vi "华为UPS2000-G-(1-3KVA)界面.vi"() -> ()   [LabVIEW 2016, in "环境动力监测库.lvlib" / "UPS库.lvlib"]
panel:
  out "Port":string
  out "IP":string
  out "x+1":u32
  in  "解除告警":bool
  out "通信":bool=TRUE
  out "串口":string
  in  "停止自检":bool
  in  "启动自检":bool
  out "UPS状态":T1
  out "电池状态":T2 {"电池状态" items=["休眠"=2, "浮充"=3, "均充"=4, "放电"=5]}
  out "UPS参数":T3 {"开机状态" items=["关机", "开机中", "开机失败", "开机完成"]}
  in  "查看型号":bool
  in  "重开串口":bool
  # "V"
  # "%"
  # "S"
  # "Ah"
  # "kVA"
  # "V"
  # "Hz"
  # "V"
  # "A"
  # "Hz"
  # "kW"
  # "kVA"
  # "%"
  # "℃"
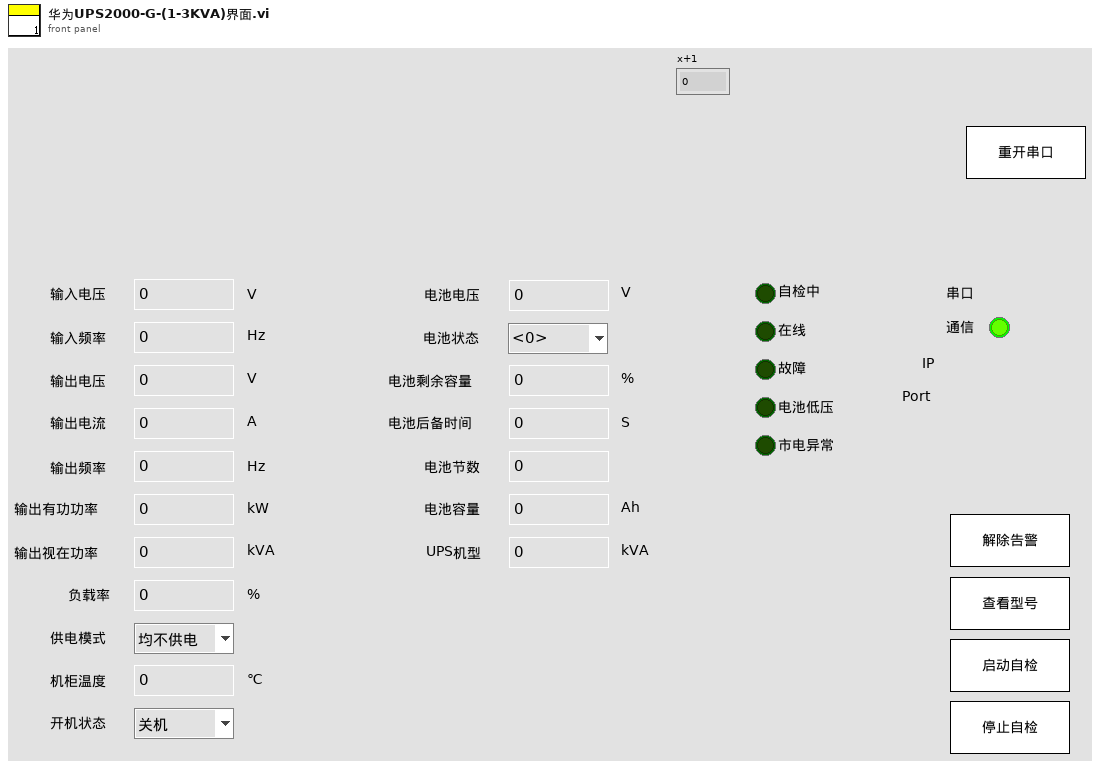
[diagram p1: front panel]
types:
  T1 = cluster{"保留":bool, "保留":bool, "自检中":bool, "在线":bool, "故障":bool, "保留":bool, "电池低压":bool, "市电异常":bool}
  T2 = cluster{"电池电压":dbl, "电池状态":u16, "电池剩余容量":u16, "电池后备时间":u32, "电池节数":u16, "电池容量":u16, "UPS机型":u16}
  T3 = cluster{"输入电压":dbl, "输入频率":dbl, "旁路电压V":dbl, "旁路频率HZ":dbl, "输出电压":dbl, "输出电流":dbl, "输出频率":dbl, "输出有功功率":dbl, "输出视在功率":dbl, "负载率":dbl, "供电模式":enum16{"均不供电", "旁路供电", "主路供电", "电池供电", "主路ECO"}, "输入制式0:单相":u16, "输出制式0:单相":u16, "机柜温度":dbl, "开机状态":u16, "UPS状态":u8}
  T4 = typedef "环境动力监测库.lvlib/UPS库.lvlib/UPS型号.ctl" = enum16{"山特UPSC1~3", "山特UPSC6~20", "华为UPS2000-G-(1-3KVA)", "Kstar"}
  T5 = cluster{"VISA resource name":refnum<visa-resource-name>, "Serial Config":cluster{"baud rate (9600)":u32, "stop bits (10: 1 bit)":u16, "parity (0:none)":enum16{"None", "Odd", "Even", "Mark", "Space"}, "data bits (8)":u16, "timeout (10sec)":u32}, "型号选择":T4, "HW-UPS-2000 MB session":refnum<class "MB_Master.lvclass">, "连接方式":enum16{"串口", "TCP"}, "IP":string, "Port":string, "低电量报警阈值":u16, "功能启用":bool}
  T6 = cluster{"输入电压V":dbl, "输入频率HZ":dbl, "旁路电压V":dbl, "旁路频率HZ":dbl, "输出电压V":dbl, "输出电流A":dbl, "输出频率HZ":dbl, "输出有功功率kW":dbl, "输出视在功率kVA":dbl, "负载率%":dbl, "供电模式":enum16{"均不供电", "旁路供电", "主路供电", "电池供电", "主路ECO"}, "输入制式0:单相":u16, "输出制式0:单相":u16, "机柜温度℃":dbl, "开机状态":u16, "UPS状态":u8}
  T7 = cluster{"电池电压V":dbl, "电池状态":u16, "电池剩余容量%":u16, "电池后备时间s":u32, "电池节数":u16, "电池容量AH":u16, "UPS机型KVA":u16}
  T8 = cluster{"市电":cluster{"状态":bool, "电压:":u16, "电流：":dbl, "详情  ":bool}, "UPS":cluster{"状态":bool, "输入电压:":sgl, "输出电压:":sgl, "电池电量:":u8, "电量":u16, "详情  ":bool}, "蓄电池12V":cluster{"状态":bool, "电压:":sgl, "电流:":sgl, "电池电量:":u8, "电量":u16, "详情  ":bool, "充电":bool, "负载":bool}, "蓄电池24V":cluster{"状态":bool, "电压:":sgl, "电流:":sgl, "电池电量:":u8, "电量":u16, "详情  ":bool, "充电":bool, "负载":bool}}
  T9 = cluster{"华为2000-G-UPS状态[0]":bool, "华为2000-G-UPS状态[1]":bool, "华为2000-G-UPS状态[2]":bool, "华为2000-G-UPS状态[3]":bool, "华为2000-G-UPS状态[4]":bool, "华为2000-G-UPS状态[5]":bool, "华为2000-G-UPS状态[6]":bool, "华为2000-G-UPS状态[7]":bool}
  T10 = enum32{"Bad", "Idle", "Run top level", "Running"}
  T11 = cluster{"漏水监测输出":cluster{"漏水监测告警":bool, "告警内容":string}, "门禁监测输出":cluster{"门禁监测告警":bool, "告警内容":string}, "门禁监测输出2":cluster{"门禁监测告警":bool, "告警内容":string}, "温湿度监测输出":cluster{"温湿度监测告警":bool, "告警内容":string}, "烟雾监测输出":cluster{"烟雾监测告警":bool, "告警内容":string}, "空调监测输出":cluster{"空调监测告警":bool, "告警内容":string}, "自动重合闸输出":cluster{"自动重合闸告警":bool, "告警内容":string}, "红外入侵输出":cluster{"红外入侵告警":bool, "告警内容":string}, "振动输出":cluster{"振动告警":bool, "告警内容":string}, "UPS输出":cluster{"UPS告警":bool, "告警内容":string}, "蓄电池输出":cluster{"蓄电池告警":bool, "告警内容":string}, "蓄电池输出2":cluster{"蓄电池告警":bool, "告警内容":string}, "GPS输出":cluster{"定位告警":bool, "告警内容":string}, "北斗输出":cluster{"定位告警":bool, "告警内容":string}, "气象输出":cluster{"气象告警":bool, "告警内容":string}, "废液输出":cluster{"废液告警":bool, "告警内容":string}, "废液输出2":cluster{"废液告警":bool, "告警内容":string}, "灭火装置输出":cluster{"灭火装置告警":bool, "告警内容":string}}
  T12 = typedef "工况数据.ctl" = cluster{"time":string, "data":cluster{"ups":cluster{"ups":cluster{"input_voltage":ext, "input_frequency":ext, "output_voltage":ext, "output_current":ext, "output_frequency":ext, "output_active_power":ext, "output_apparent_power":ext, "load_rate":ext, "cabinet_temperature":ext, "battery_voltage":ext, "remaining_battery_capacity":ext, "power_on_status":string, "power_supply_mode":string, "fault":bool, "battery_low_voltage":bool, "mains_supply_abnormality":bool}, "启用":bool}, "air_conditioner":cluster{"air_conditioner":cluster{"cabinet_temperature":ext, "air_supply_temperature":ext, "voltage":ext, "current":ext, "compressor_status":string, "Internal_fan_status":string, "external_fan_status":string, "heating_state":string, "refrigeration_state":bool, "high_temperature_alarm":bool, "low_temperature_alarm":bool, "heater_fault":bool, "temperature_sensor_fault":bool, "high_voltage_alarm":bool, "low_voltage_alarm":bool, "refrigeration_start_point":ext, "refrigeration_sensitive_point":ext, "heating_start_point":ext, "heating_sensitive_point":ext, "high_temperature_alarm_point":ext, "low_temperature_alarm_point":ext}, "启用":bool}, "smoke_sensor":cluster{"smoke_sensor":cluster{"trigger_alarm":bool}, "启用":bool}, "water_immersion_sensor":cluster{"water_immersion_sensor":cluster{"trigger_alarm":bool}, "启用":bool}, "temperature_and_humidity_sensor":cluster{"temperature_and_humidity_sensor":cluster{"current_temperature":ext, "current_humidity":ext, "room_temperature_alarm":bool, "humidity_alarm":bool}, "启用":bool}, "gps":cluster{"gps":cluster{"current_longitude":ext, "current_latitude":ext, "launch_longitude":ext, "launch_latitude":ext, "shift_alarm":bool}, "启用":bool}, "solar_controller":cluster{"solar_controller":cluster{"array_voltage":ext, "array_current":ext, "generating_power":ext, "battery_voltage":dbl, "battery_current":ext, "ceiling_voltage":ext, "minimum_voltage":ext, "battery_temperature":ext, "remaining_battery_capacity":ext, "load_voltage":ext, "load_current":ext, "load_power":ext, "equipment_temperature":ext, "accumulated_electricity_consumption_of_the_day":ext, "accumulated_electricity_consumption_of_the_current_month":ext, "accumulated_electricity_consumption_in_the_current_year":ext, "total_accumulated_power_consumption":ext, "accumulated_charging_capacity_of_the_day":ext, "accumulated_charging_amount_of_the_current_month":ext, "accumulated_charging_capacity_of_the_current_year":ext, "total_cumulative_charge":ext}, "启用":bool}, "solar_controller_2":cluster{"solar_controller_2":cluster{"array_voltage":ext, "array_current":ext, "generating_power":ext, "battery_voltage":dbl, "battery_current":ext, "ceiling_voltage":ext, "minimum_voltage":ext, "battery_temperature":ext, "remaining_battery_capacity":ext, "load_voltage":ext, "load_current":ext, "load_power":ext, "equipment_temperature":ext, "accumulated_electricity_consumption_of_the_day":ext, "accumulated_electricity_consumption_of_the_current_month":ext, "accumulated_electricity_consumption_in_the_current_year":ext, "total_accumulated_power_consumption":ext, "accumulated_charging_capacity_of_the_day":ext, "accumulated_charging_amount_of_the_current_month":ext, "accumulated_charging_capacity_of_the_current_year":ext, "total_cumulative_charge":ext}, "启用":bool}, "NH3":cluster{"NH3":cluster{"F0":ext, "F1":ext, "syringe_temperature":ext, "alarm_step":dbl, "X0":ext}, "启用":bool}, "TP":cluster{"TP":cluster{"F0":ext, "F1":ext, "F2":ext, "F3":ext, "digestion_temperature":ext, "constant_temperature":ext, "syringe_temperature":ext, "alarm_step":dbl, "X0":ext}, "启用":bool}, "TN":cluster{"TN":cluster{"F0":ext, "F1":ext, "F2":ext, "F3":ext, "F4":ext, "F5":ext, "F6":ext, "F7":ext, "digestion_temperature":ext, "constant_temperature":ext, "syringe_temperature":ext, "alarm_step":dbl, "X0":ext}, "启用":bool}, "CODMn":cluster{"CODMn":cluster{"temperature_curve":ext[], "titration_curve":ext[], "F0":ext, "F1":ext, "F2":ext, "F3":ext, "F4":ext, "F5":ext, "A":ext, "B":ext, "K":ext}, "启用":bool}, "CODCr":cluster{"CODCr":cluster{"temperature_curve":ext[], "F0":ext, "F1":ext, "reagent_sensor":ext}, "启用":bool}}}
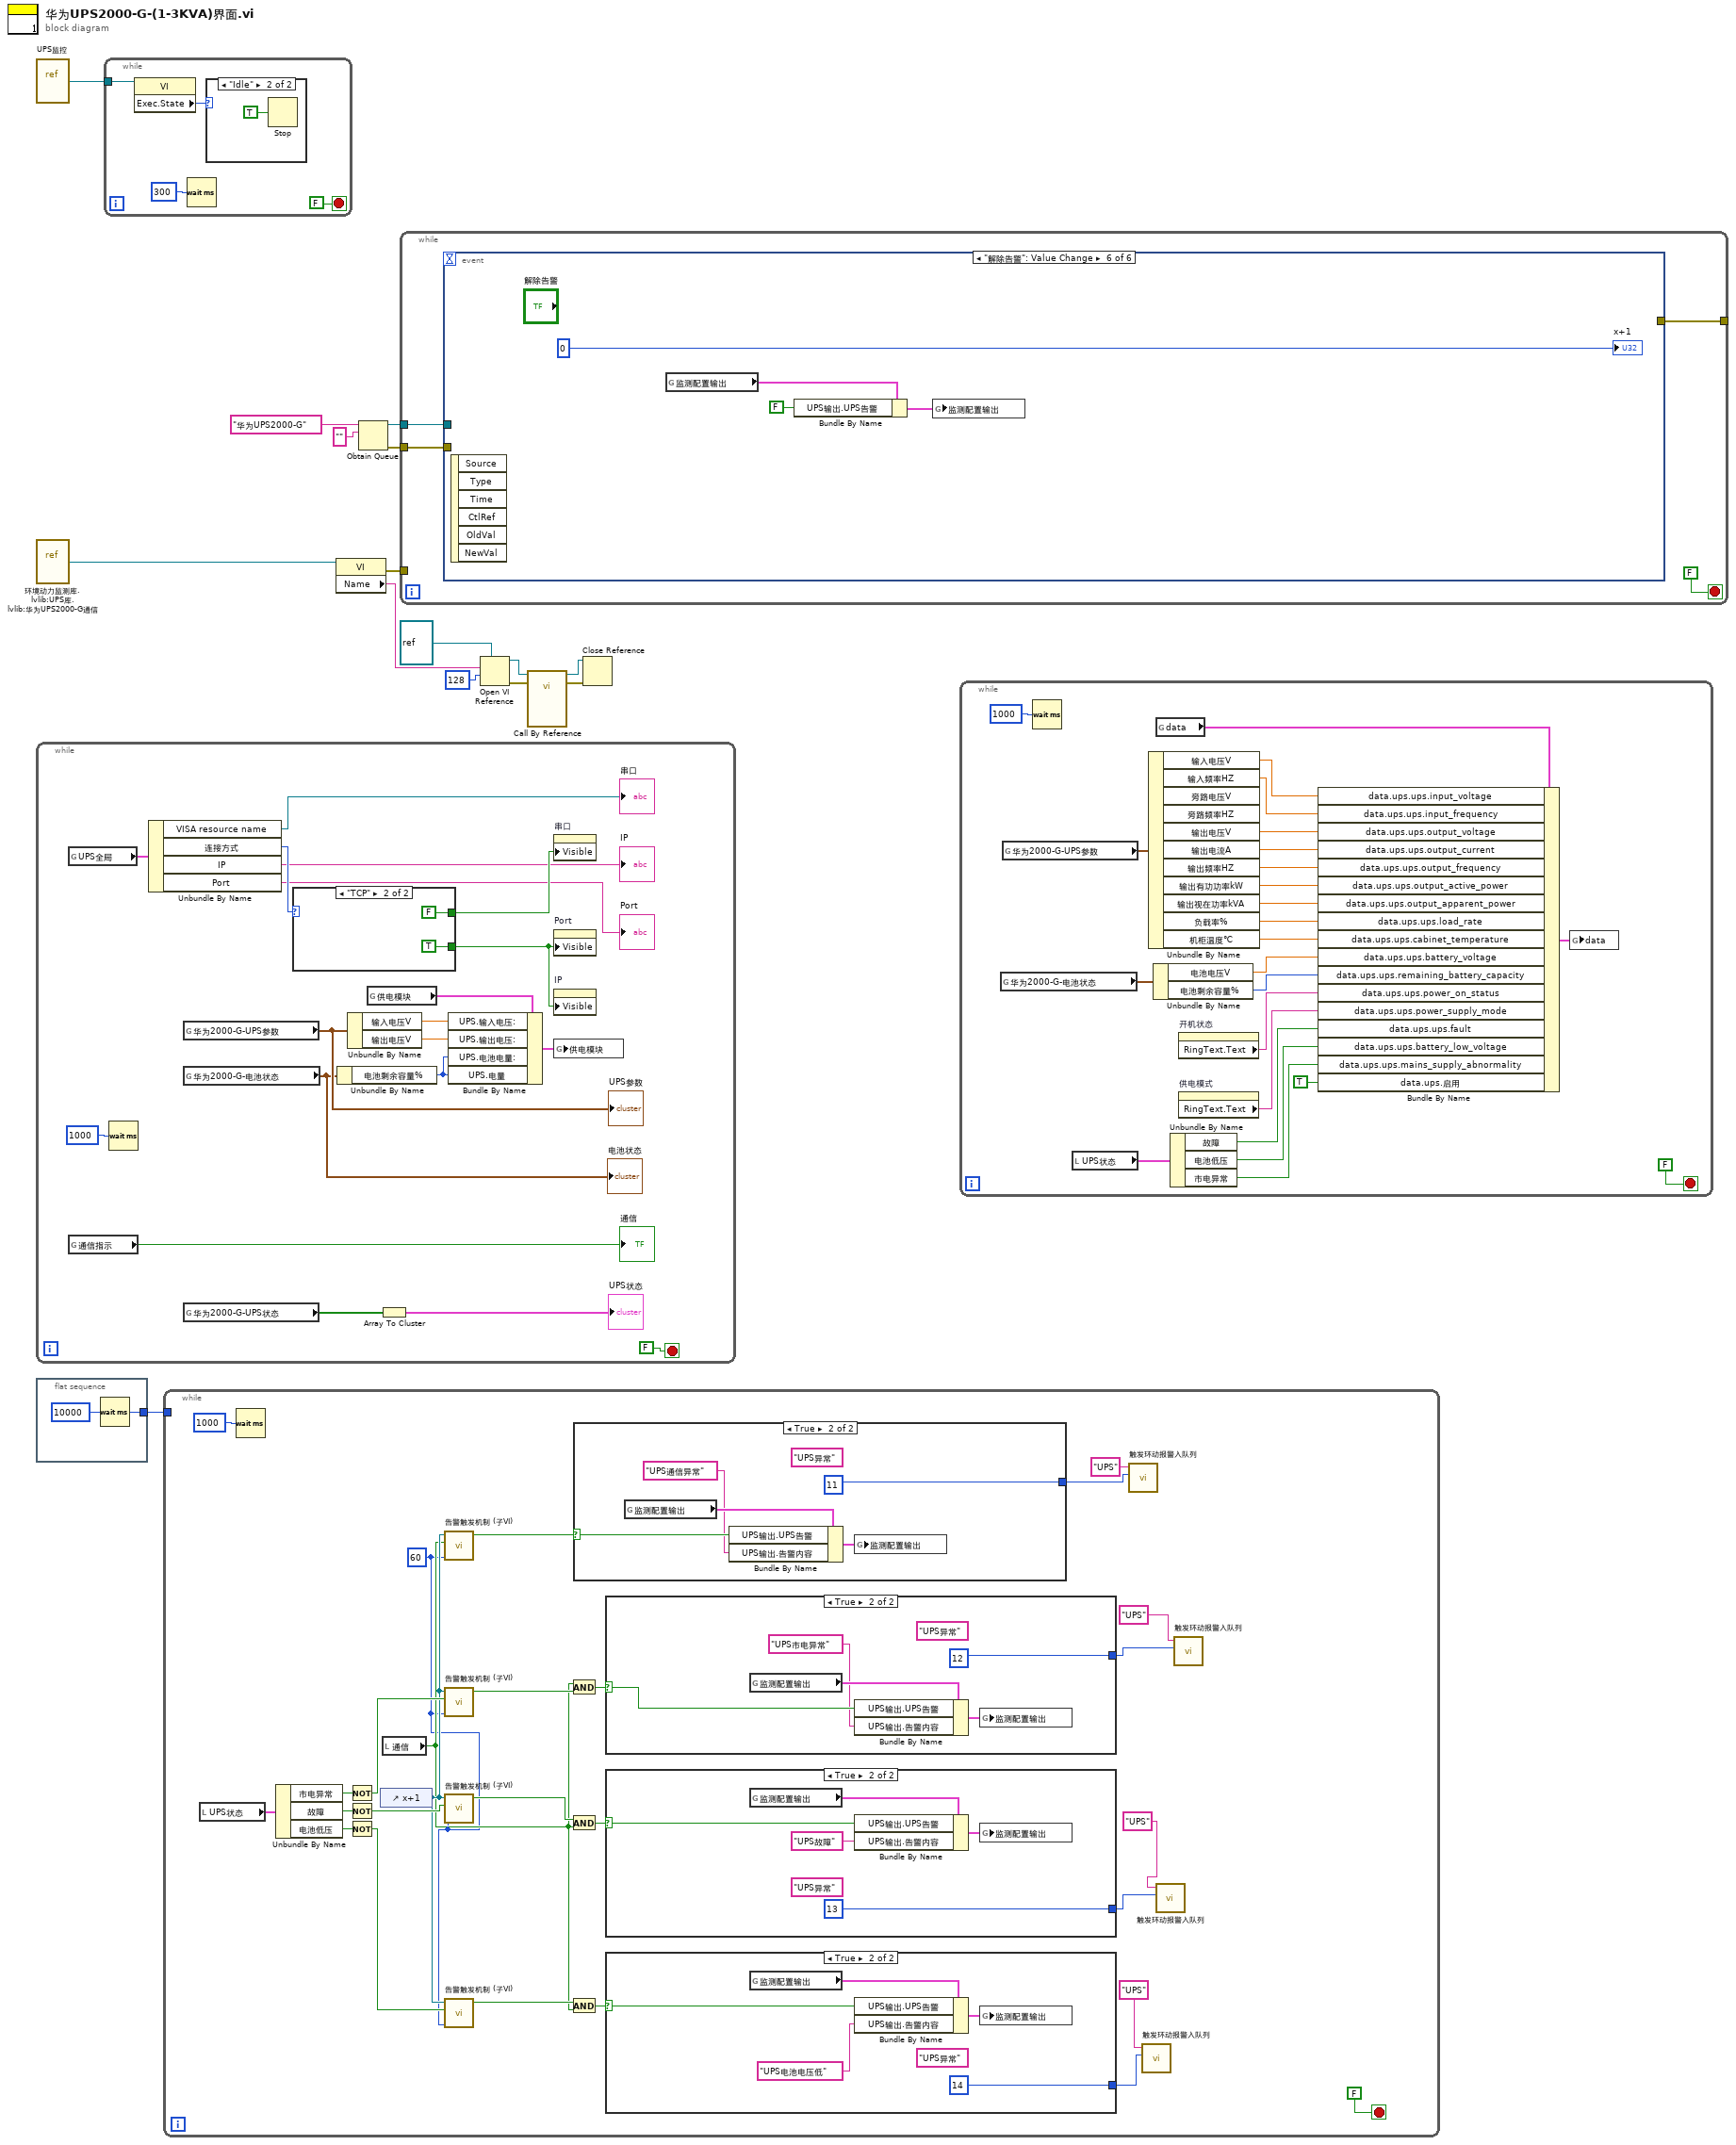
[diagram p0: block diagram]
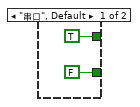
[diagram p7: hidden frame]
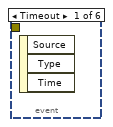
[diagram p8: hidden frame]
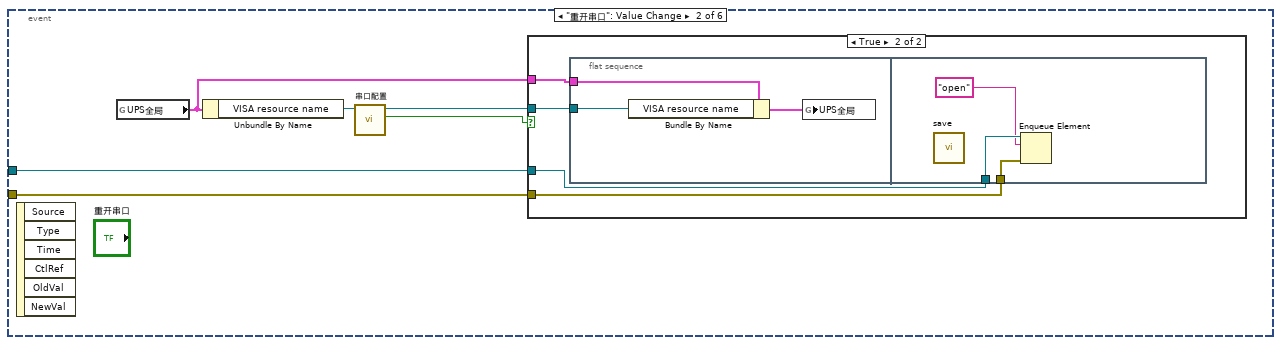
[diagram p9: hidden frame]
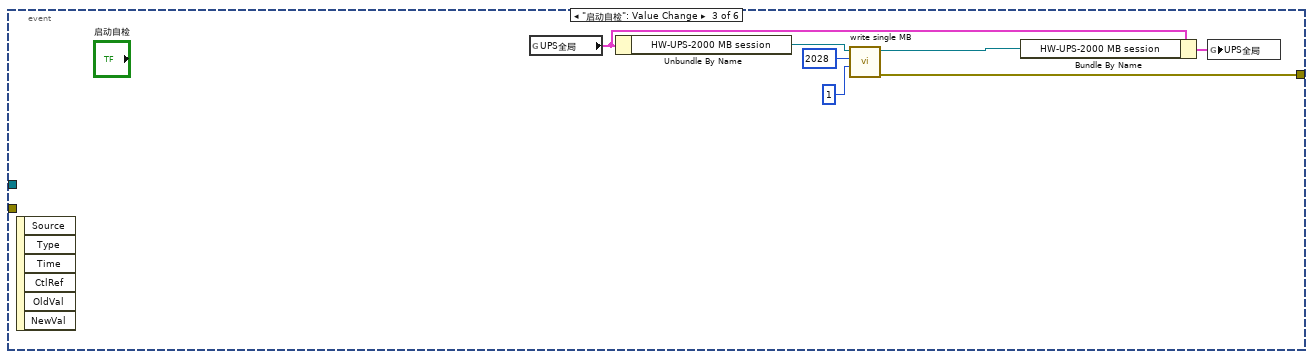
[diagram p11: hidden frame]
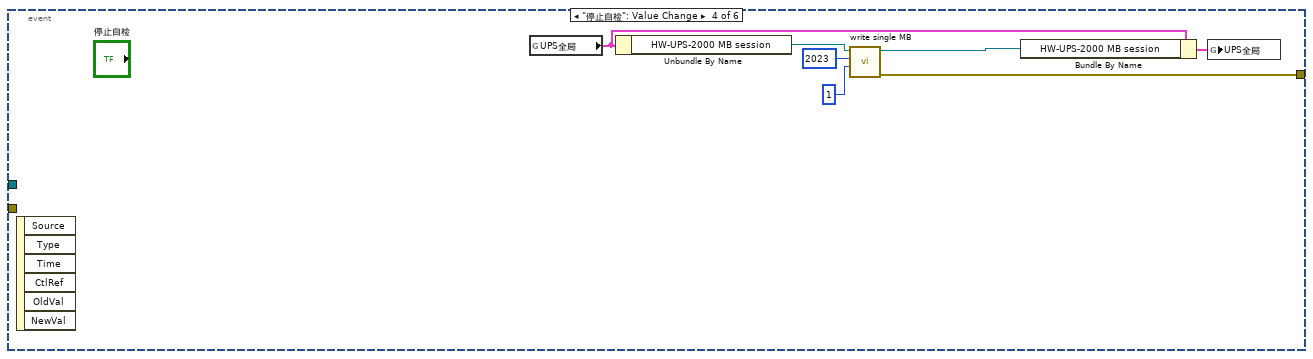
[diagram p12: hidden frame]
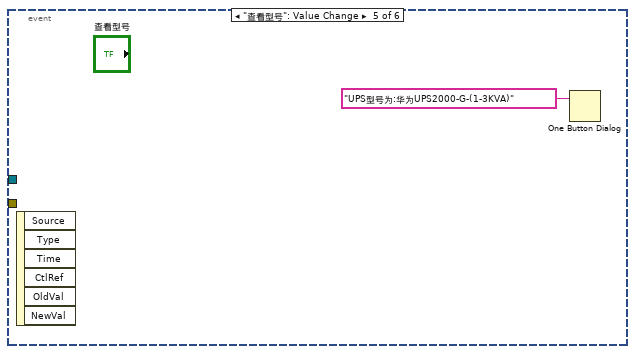
[diagram p13: hidden frame]
diagram:
  n1 = vi-ref "UPS监控.vi"() -> (w2:refnum<vi>)
  n2 = vi-ref "环境动力监测库.lvlib:UPS库.lvlib:华为UPS2000-G通信.vi"() -> (w8:refnum<vi>)
  n3 = while {
    stop <- FALSE stop-if-true
    n4 = global read "断电保存全局变量.vi" "UPS全局"() -> (w20:T5)
    n5 = global read "UPS内部交互全局.vi" "通信指示"() -> (→"通信":bool)
    n6 = Wait (ms)(milliseconds to wait=u32 1000 ("等待时间（毫秒）")) -> ()  [unwired: 1 out]
    n7 = Unbundle By Name(w20) -> ("VISA resource name"=→"串口":refnum<visa-resource-name>, "连接方式"=w18:enum16{"串口", "TCP"}, "IP"=→"IP":string, "Port"=→"Port":string)
    n8 = global read "UPS内部交互全局.vi" "华为2000-G-UPS参数"() -> (w29:T6)
    "UPS参数" <- w29
    n9 = global read "UPS内部交互全局.vi" "华为2000-G-电池状态"() -> (w26:T7)
    "电池状态" <- w26
    n10 = global read "UPS内部交互全局.vi" "华为2000-G-UPS状态"() -> (w24:bool[])
    n11 = case shown="\"TCP\"" w18 {
      tunnel: [TRUE FALSE] -> w22
      tunnel: [FALSE TRUE] -> w21
      frame "串口", Default {
      }
      frame "TCP" {
      }
    }
    n12 = Unbundle By Name(w26) -> ("电池剩余容量%"=w25:u16)
    n13 = Unbundle By Name(w29) -> ("输入电压V"=w28:dbl, "输出电压V"=w27:dbl)
    n14 = global read "内部交互全局变量.vi" "供电模块"() -> (w31:T8)
    n15 = Array To Cluster(array=w24) -> (cluster=→"UPS状态":T9)
    n16 = Bundle By Name(cluster=w31, "UPS.输入电压:"=w28, "UPS.输出电压:"=w27, "UPS.电池电量:"=w25, "UPS.电量"=w25) -> (w30:T8)
    n17 = property on="串口" class="Str"("Visible"=w22) -> ()  [unwired: 2 in, 2 out]
    n18 = property on="Port" class="Str"("Visible"=w21) -> ()  [unwired: 2 in, 2 out]
    n19 = property on="IP" class="Str"("Visible"=w21) -> ()  [unwired: 2 in, 2 out]
    n20 = global write "内部交互全局变量.vi" "供电模块"(w30) -> ()
  }
  n21 = flat-sequence {
    tunnel: [w39] -> w1
    frame #0 {
      n22 = Wait (ms)(milliseconds to wait=u32 10000 ("等待时间（毫秒）")) -> (millisecond timer value=w39:u32)
    }
  }
  n23 = while {
    tunnel: w2 -> [w44]
    stop <- FALSE stop-if-true
    n24 = property class="VI"(reference=w44) -> ("Exec.State"=w43:T10)  [unwired: 1 in, 2 out]
    n25 = Wait (ms)(milliseconds to wait=u32 300 ("等待时间（毫秒）")) -> ()  [unwired: 1 out]
    n26 = case shown="\"Idle\"" w43 {
      frame "Bad", Default {
      }
      frame "Idle" {
        n27 = Stop(stop? (T)=TRUE ("停止？(T)")) -> ()
      }
    }
  }
  n28 = while {
    tunnel: w1 -> [_]
    stop <- FALSE stop-if-true
    w54 = u32 60 ("信号持续时间")
    n29 = local read "UPS状态"() -> (w70:T1)
    n30 = Wait (ms)(milliseconds to wait=u32 1000 ("等待时间（毫秒）")) -> ()  [unwired: 1 out]
    n31 = Unbundle By Name(w70) -> ("市电异常"=w68:bool, "故障"=w65:bool, "电池低压"=w62:bool)
    n32 = Not(x=w68) -> (.not. x?=w69:bool)
    n33 = Not(x=w65) -> (.not. x?=w66:bool)
    n34 = Not(x=w62) -> (.not. x?=w63:bool)
    n35 = control-ref of="x+1"() -> (w60:refnum<vi>)
    n36 = local read "通信"() -> (w56:bool)
    n37 = call "告警触发机制 (子VI).vi"("信号持续时间"=w54, "状态输出真-正常"=w56, "Digital输入"=w60) -> ("触发告警"=w55:bool)  [unwired: 6 in, 2 out]
    n38 = call "告警触发机制 (子VI).vi"("信号持续时间"=w54, "状态输出真-正常"=w69, "Digital输入"=w60) -> ("触发告警"=w67:bool)  [unwired: 6 in, 2 out]
    n39 = call "告警触发机制 (子VI).vi"("信号持续时间"=w54, "状态输出真-正常"=w66, "Digital输入"=w60) -> ("触发告警"=w64:bool)  [unwired: 6 in, 2 out]
    n40 = call "告警触发机制 (子VI).vi"("信号持续时间"=w54, "状态输出真-正常"=w63, "Digital输入"=w60) -> ("触发告警"=w61:bool)  [unwired: 6 in, 2 out]
    n41 = And(x=w56, y=w67) -> (x .and. y?=w59:bool)
    n42 = And(x=w64, y=w56) -> (x .and. y?=w58:bool)
    n43 = And(x=w61, y=w56) -> (x .and. y?=w57:bool)
    n44 = case shown="True" w55 {
      selector: w55 -> [_ w82]
      tunnel: [_ 11 ("code")] -> w52
      frame False {
      }
      frame True {
        (unwired) "UPS异常" ("设备")
        n45 = global read "内部交互全局变量.vi" "监测配置输出"() -> (w80:T11)
        n46 = Bundle By Name(cluster=w80, "UPS输出.UPS告警"=w82, "UPS输出.告警内容"="UPS通信异常" ("报警内容")) -> (w81:T11)
        n47 = global write "内部交互全局变量.vi" "监测配置输出"(w81) -> ()
      }
    }
    n48 = case shown="True" w59 {
      selector: w59 -> [_ w92]
      tunnel: [_ 12 ("code")] -> w50
      frame False {
      }
      frame True {
        (unwired) "UPS异常" ("设备")
        n49 = global read "内部交互全局变量.vi" "监测配置输出"() -> (w91:T11)
        n50 = Bundle By Name(cluster=w91, "UPS输出.UPS告警"=w92, "UPS输出.告警内容"="UPS市电异常" ("报警内容")) -> (w90:T11)
        n51 = global write "内部交互全局变量.vi" "监测配置输出"(w90) -> ()
      }
    }
    n52 = case shown="True" w58 {
      selector: w58 -> [_ w77]
      tunnel: [_ 13 ("code")] -> w48
      frame False {
      }
      frame True {
        (unwired) "UPS异常" ("设备")
        n53 = global read "内部交互全局变量.vi" "监测配置输出"() -> (w76:T11)
        n54 = Bundle By Name(cluster=w76, "UPS输出.UPS告警"=w77, "UPS输出.告警内容"="UPS故障" ("报警内容")) -> (w75:T11)
        n55 = global write "内部交互全局变量.vi" "监测配置输出"(w75) -> ()
      }
    }
    n56 = case shown="True" w57 {
      selector: w57 -> [_ w87]
      tunnel: [_ 14 ("code")] -> w47
      frame False {
      }
      frame True {
        (unwired) "UPS异常" ("设备")
        n57 = global read "内部交互全局变量.vi" "监测配置输出"() -> (w86:T11)
        n58 = Bundle By Name(cluster=w86, "UPS输出.UPS告警"=w87, "UPS输出.告警内容"="UPS电池电压低" ("报警内容")) -> (w85:T11)
        n59 = global write "内部交互全局变量.vi" "监测配置输出"(w85) -> ()
      }
    }
    n60 = call "触发环动报警入队列.vi"("code"=w52, "元器件"="UPS") -> ()  [unwired: 10 in]
    n61 = call "触发环动报警入队列.vi"("code"=w47, "元器件"="UPS") -> ()  [unwired: 10 in]
    n62 = call "触发环动报警入队列.vi"("code"=w48, "元器件"="UPS") -> ()  [unwired: 10 in]
    n63 = call "触发环动报警入队列.vi"("code"=w50, "元器件"="UPS") -> ()  [unwired: 10 in]
  }
  n64 = property class="VI"(reference=w8) -> (error out=w4:errorcluster, "Name"=w9:string)  [unwired: 1 in, 1 out]
  n65 = Obtain Queue(name (unnamed)="华为UPS2000-G" ("名称（未命名）"), element data type="") -> (queue out=w6:refnum<queue>, error out=w5:errorcluster)  [unwired: 3 in, 1 out]
  n66 = while {
    tunnel: w5 -> [w95]
    tunnel: w6 -> [w94]
    tunnel: w4 -> [_]
    tunnel: [w93] -> _
    stop <- FALSE stop-if-true
    n67 = event shown="[5] \"解除告警\": Value Change" {
      selector: _ -> [_ _ _ _ _ _]
      dyn-events: _ -> [_ _ _ _ _ _]
      timeout: _ -> [_ _ _ _ _ _]
      tunnel: w95 -> [_ w99 _ _ _ _]
      tunnel: w94 -> [_ w100 _ _ _ _]
      tunnel: [_ _ w117 w124 _ _] -> w93
      event Timeout {
        n68 = event-data() -> ()  [unwired: 1 in, 3 out]
      }
      event "重开串口": Value Change {
        n69 = event-data() -> ()  [unwired: 1 in, 6 out]
        n70 = global read "断电保存全局变量.vi" "UPS全局"() -> (w97:T5)
        n71 = Unbundle By Name(w97) -> ("VISA resource name"=w98:refnum<visa-resource-name>)
        n72 = call "串口配置.vi"("请选择串口:"=w98) -> ("确认 2"=w102:bool, "请选择串口: 2"=w101:refnum<visa-resource-name>)  [unwired: 9 in]
        n73 = case shown="True" w102 {
          tunnel: w101 -> [_ w106]
          tunnel: w100 -> [_ w105]
          tunnel: w99 -> [_ w104]
          tunnel: w97 -> [_ w103]
          frame False {
          }
          frame True {
            n74 = flat-sequence {
              tunnel: w106 -> [w109]
              tunnel: w103 -> [w108]
              tunnel: w105 -> [w112]
              tunnel: w104 -> [w111]
              frame #0 {
                n75 = Bundle By Name(cluster=w108, "VISA resource name"=w109) -> (w107:T5)
                n76 = global write "断电保存全局变量.vi" "UPS全局"(w107) -> ()
              }
              frame #1 {
                n77 = call "save.vi"() -> ()  [unwired: 11 in, 1 out]
                n78 = Enqueue Element(queue=w112, element="open" ("元素"), error in (no error)=w111) -> ()  [unwired: 1 in, 3 out]
              }
            }
          }
        }
      }
      event "启动自检": Value Change {
        n79 = event-data() -> ()  [unwired: 1 in, 6 out]
        n80 = global read "断电保存全局变量.vi" "UPS全局"() -> (w113:T5)
        n81 = Unbundle By Name(w113) -> ("HW-UPS-2000 MB session"=w116:refnum<class "MB_Master.lvclass">)
        n82 = call "write single MB.vi"("value"=u16 1, "address"=u16 2028, "MB session in"=w116) -> ("error out"=w117:errorcluster, "MB session out"=w114:refnum<class "MB_Master.lvclass">)  [unwired: 7 in]
        n83 = Bundle By Name(cluster=w113, "HW-UPS-2000 MB session"=w114) -> (w115:T5)
        n84 = global write "断电保存全局变量.vi" "UPS全局"(w115) -> ()
      }
      event "停止自检": Value Change {
        n85 = event-data() -> ()  [unwired: 1 in, 6 out]
        n86 = global read "断电保存全局变量.vi" "UPS全局"() -> (w120:T5)
        n87 = Unbundle By Name(w120) -> ("HW-UPS-2000 MB session"=w123:refnum<class "MB_Master.lvclass">)
        n88 = call "write single MB.vi"("value"=u16 1, "address"=u16 2023, "MB session in"=w123) -> ("error out"=w124:errorcluster, "MB session out"=w121:refnum<class "MB_Master.lvclass">)  [unwired: 7 in]
        n89 = Bundle By Name(cluster=w120, "HW-UPS-2000 MB session"=w121) -> (w122:T5)
        n90 = global write "断电保存全局变量.vi" "UPS全局"(w122) -> ()
      }
      event "查看型号": Value Change {
        n91 = event-data() -> ()  [unwired: 1 in, 6 out]
        n92 = One Button Dialog(message="UPS型号为:华为UPS2000-G-(1-3KVA)" ("消息")) -> ()  [unwired: 1 in, 1 out]
      }
      event "解除告警": Value Change {
        n93 = event-data() -> ()  [unwired: 1 in, 6 out]
        n94 = global read "内部交互全局变量.vi" "监测配置输出"() -> (w129:T11)
        n95 = Bundle By Name(cluster=w129, "UPS输出.UPS告警"=FALSE) -> (w128:T11)
        n96 = global write "内部交互全局变量.vi" "监测配置输出"(w128) -> ()
        "x+1" <- u32 0 ("x+1")
      }
    }
  }
  n97 = Open VI Reference(type specifier VI Refnum (for type only)=refnum<vi> refnum, vi path=w9, options=128 ("选项")) -> (vi reference=w11:refnum<vi>, error out=w13:errorcluster)  [unwired: 3 in]
  n98 = call-by-ref "?"(reference=w11, error in=w13) -> (reference out=w15:refnum<vi>, error out=w14:errorcluster)  [unwired: 12 in]
  n99 = Close Reference(reference=w15, error in (no error)=w14) -> ()  [unwired: 1 out]
  n100 = while {
    stop <- FALSE stop-if-true
    n101 = global read "UPS内部交互全局.vi" "华为2000-G-电池状态"() -> (w150:T7)
    n102 = global read "UPS内部交互全局.vi" "华为2000-G-UPS参数"() -> (w152:T6)
    n103 = Wait (ms)(milliseconds to wait=u32 1000 ("等待时间（毫秒）")) -> ()  [unwired: 1 out]
    n104 = local read "UPS状态"() -> (w136:T1)
    n105 = Unbundle By Name(w152) -> ("输入电压V"=w149:dbl, "输入频率HZ"=w148:dbl, "输出电压V"=w147:dbl, "输出电流A"=w146:dbl, "输出频率HZ"=w145:dbl, "输出有功功率kW"=w144:dbl, "输出视在功率kVA"=w143:dbl, "负载率%"=w142:dbl, "机柜温度℃"=w141:dbl)  [unwired: 2 out]
    n106 = Unbundle By Name(w150) -> ("电池电压V"=w140:dbl, "电池剩余容量%"=w139:u16)
    n107 = global read "工况数据接口全局.vi" "data"() -> (w155:T12)
    n108 = Unbundle By Name(w136) -> ("故障"=w135:bool, "电池低压"=w134:bool, "市电异常"=w133:bool)
    n109 = property on="开机状态" class="Ring (strict)"() -> ("RingText.Text"=w138:string)  [unwired: 2 in, 2 out]
    n110 = property on="供电模式" class="Enum (strict)"() -> ("RingText.Text"=w137:string)  [unwired: 2 in, 2 out]
    n111 = Bundle By Name(cluster=w155, "data.ups.ups.input_voltage"=w149, "data.ups.ups.input_frequency"=w148, "data.ups.ups.output_voltage"=w147, "data.ups.ups.output_current"=w146, "data.ups.ups.output_frequency"=w145, "data.ups.ups.output_active_power"=w144, "data.ups.ups.output_apparent_power"=w143, "data.ups.ups.load_rate"=w142, "data.ups.ups.cabinet_temperature"=w141, "data.ups.ups.battery_voltage"=w140, "data.ups.ups.remaining_battery_capacity"=w139, "data.ups.ups.power_on_status"=w138, "data.ups.ups.power_supply_mode"=w137, "data.ups.ups.fault"=w135, "data.ups.ups.battery_low_voltage"=w134, "data.ups.ups.mains_supply_abnormality"=w133, "data.ups.启用"=TRUE) -> (w151:T12)
    n112 = global write "工况数据接口全局.vi" "data"(w151) -> ()
  }
